vi "Component Loader.Load.Class.vi"(8 "error in (no error)":errorcluster, 10 "class path":path, 11 "Component Loader in":refnum<class "Component Loader.lvclass">) -> (0 "error out":errorcluster, 2 "object":refnum<class>, 3 "Component Loader out":refnum<class "Component Loader.lvclass">)   [LabVIEW 2017, in "DSF Core.lvlib" / "Component Loader.lvclass"]
uses:
  Component Loader.lvclass
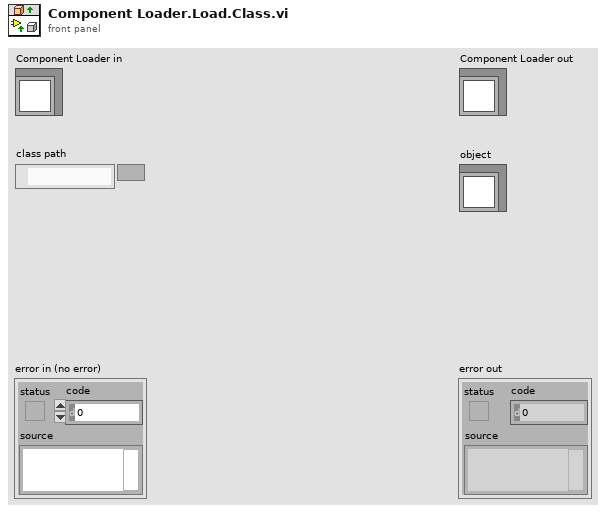
[diagram p1: front panel]
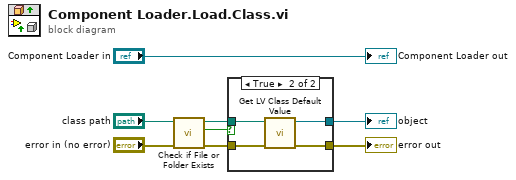
[diagram p0: block diagram]
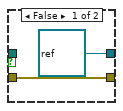
[diagram p2: hidden frame]
diagram:
  n1 = call <vilib>:"Check if File or Folder Exists.vi"("error in (no error)"="error in (no error)", "path"="class path") -> ("error out"=w6:errorcluster, "file or folder exists?"=w7:bool, "dup path"=w5:path)  [unwired: 7 in]
  n2 = case shown="True" w7 {
    tunnel: w6 -> [w9 w14]
    tunnel: w5 -> [_ w13]
    tunnel: [refnum<class> refnum ("object") w12] -> w2
    tunnel: [w9 w11] -> w1
    frame False {
    }
    frame True {
      n3 = call <vilib>:"Get LV Class Default Value.vi"("error in (no error)"=w14, "class path"=w13) -> ("error out"=w11:errorcluster, "object"=w12:refnum<class>)  [unwired: 8 in]
    }
  }
  "error out" <- w1
  "object" <- w2
  "Component Loader out" <- "Component Loader in"
